vi "add action.vi"(6 "user event":T1, 8 "error in":errorcluster, 9 "channel list":refnum<vi>, 10 "engine configuration in":refnum<class "engine configuration.lvclass">, 11 "io configuration in":refnum<class "io configuration.lvclass">) -> (0 "error out":errorcluster, 2 "engine configuration out":refnum<class "engine configuration.lvclass">, 3 "io configuration out":refnum<class "io configuration.lvclass">)   [LabVIEW 2014, in "io editor node.lvclass"]
uses:
  io editor node.lvclass
  <vilib>/NI/Configuration Framework/Controls/EventCluster.ctl
  <vilib>/NI/Configuration Framework/NISE_CEF_TreeControl.lvlib
  <vilib>/NI/Tag Bus Module Framework/channel/TBM channel.lvclass
  <vilib>/NI/Configuration Framework/serializable configuration/NISE_CEF_serializable configuration.lvclass
  configuration/io configuration.lvclass
  <vilib>/NI/Module Execution Interface/Engine Configuration/engine configuration.lvclass
  <vilib>/NI/Configuration Framework/Node/UserEventRef.ctl
  <vilib>/NI/Configuration Framework/Node/NISE_CEF_Node.lvclass
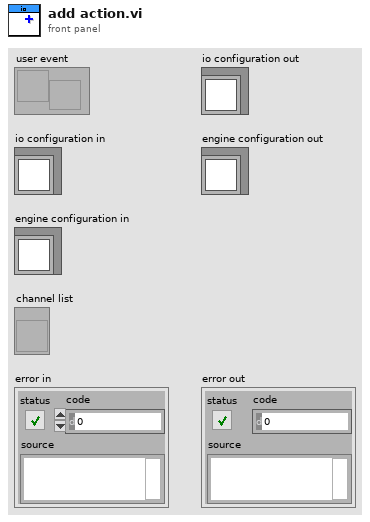
[diagram p1: front panel]
types:
  T1 = typedef "NISE_CEF_Node.lvclass/UserEventRef.ctl" = refnum<user-event>
  T2 = typedef "io editor node.lvclass/table line.ctl" = cluster{"channel":refnum<class "TBM channel.lvclass">, "tag name":string}
  T3 = typedef "NISE_CEF_TreeControl.lvlib/EventCluster.ctl" = cluster{"command":string, "data":string}
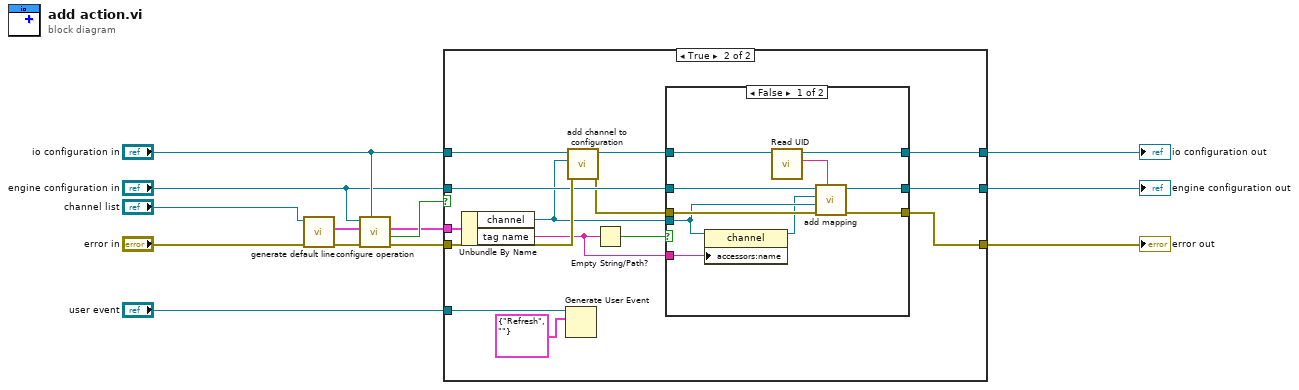
[diagram p0: block diagram]
diagram:
  n1 = call "generate default line.vi"("error in"="error in", "operations table"="channel list") -> ("error out"=w3:errorcluster, "line"=w2:T2)  [unwired: 8 in]
  n2 = call "configure operation.vi"("tag bus configurable plugin module configuration"="io configuration in", "error in"=w3, "line item in"=w2, "engine configuration"="engine configuration in") -> ("error out"=w5:errorcluster, "success"=w6:bool, "line item out"=w4:T2)  [unwired: 4 in, 1 out]
  n3 = case shown="True" w6 {
    tunnel: [w16 w19] -> w1
    tunnel: w5 -> [w16 w28]
    tunnel: "engine configuration in" -> [w15 w26]
    tunnel: w4 -> [_ w29]
    tunnel: "io configuration in" -> [w14 w30]
    tunnel: [w15 w25] -> w13
    tunnel: [w14 w20] -> w12
    tunnel: "user event" -> [_ w18]
    frame False {
    }
    frame True {
      n4 = Unbundle By Name(w29) -> ("channel"=w23:refnum<class "TBM channel.lvclass">, "tag name"=w22:string)
      n5 = Generate User Event(user event=w18, event data cluster=T3 {"command"="Refresh", "data"=""} ("event data")) -> ()  [unwired: 2 in, 2 out]
      n6 = call "add channel to configuration.vi"("error in"=w28, "channel"=w23, "io configuration in"=w30) -> ("error out"=w24:errorcluster, "io configuration out"=w21:refnum<class "io configuration.lvclass">)  [unwired: 7 in]
      n7 = Empty String/Path?(string/path=w22) -> (empty?=w27:bool)
      n8 = case shown="False" w27 {
        tunnel: w26 -> [w40 w43]
        tunnel: [w39 w43] -> w25
        tunnel: w24 -> [w38 w42]
        tunnel: w23 -> [w37 _]
        tunnel: w22 -> [w36 _]
        tunnel: [w34 w42] -> w19
        tunnel: w21 -> [w33 w41]
        tunnel: [w32 w41] -> w20
        frame False {
          n9 = property class="channel"(reference=w37, "accessors:name"=w36) -> (reference out=w35:refnum<class "TBM channel.lvclass">)  [unwired: 1 in, 1 out]
          n10 = call <vilib>:"Read UID.vi"("configuration in"=w33) -> ("instance id"=w31:string, "configuration out"=w32:refnum<class "io configuration.lvclass">)  [unwired: 8 in, 1 out]
          n11 = call-dynamic "add mapping.vi"("owner ID"=w31, "error in"=w38, "channel"=w37, "tag descriptor"=w35, "engine configuration"=w40) -> ("error out"=w34:errorcluster, "engine configuration out"=w39:refnum<class "engine configuration.lvclass">)  [unwired: 5 in]
        }
        frame True {
        }
      }
    }
  }
  "engine configuration out" <- w13
  "io configuration out" <- w12
  "error out" <- w1
